vi "ExSubToggleBackGrnd.vi"(2 "error in (no error)":errorcluster, 3 "Camera Handle":u32) -> (0 "error out":errorcluster, 1 "Camera Handle":u32)   [LabVIEW 2010]
uses:
  GlobalIBackImgHndl.vi
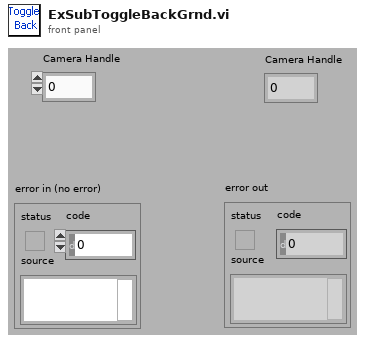
[diagram p1: front panel]
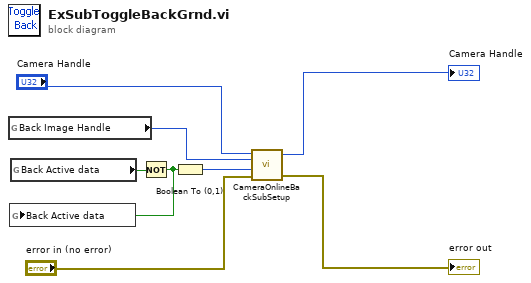
[diagram p0: block diagram]
diagram:
  n1 = global read "GlobalIBackImgHndl.vi" "Back Image Handle"() -> (w4:u32)
  n2 = global read "GlobalIBackImgHndl.vi" "Back Active data"() -> (w8:bool)
  n3 = Not(x=w8) -> (.not. x?=w1:bool)
  n4 = global write "GlobalIBackImgHndl.vi" "Back Active data"(w1) -> ()
  n5 = Boolean To (0,1)(Boolean=w1) -> (0, 1=w7:i16)
  n6 = call <userlib>:"CameraOnlineBackSubSetup.vi"("error in"="error in (no error)", "Background Flag"=w7, "Background Image Handle"=w4, "Camera Handle"="Camera Handle") -> ("error out"=→"error out":errorcluster, "Camera Handle"=→"Camera Handle":u32)  [unwired: 1 out]
